vi "Get System Property.vi"   [LabVIEW 2020, in "SLSC.lvlib"]
uses:
  <vilib>/SLSC/SLSC.lvlib
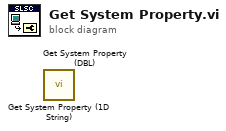
[diagram p0: block diagram]
diagram:
  n1 = call <vilib>:"Get System Property (1D String).vi"() -> ()  [unwired: 13 in, 3 out]
  n2 = call <vilib>:"Get System Property (DBL).vi"() -> ()  [unwired: 13 in, 3 out]
